vi "BS find all the buoys.vi"(0 "Image Src":T1, 1 "error in":errorcluster) -> (2 "Buoy Array":cluster{i16, i16}[](array[cluster]), 3 "Buoys found?":bool, 4 "error out":errorcluster)   [LabVIEW 2012]
doc: "This VI finds all the buoys and places there location into a 2D array. A valid flag is posted if completed."
uses:
  <vilib>/vision/Image Controls.llb/IMAQ Image.ctl
  <vilib>/vision/NI_Vision_Development_Module.lvlib
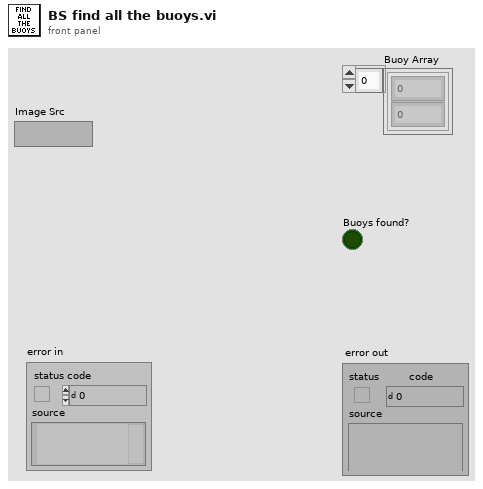
[diagram p1: front panel]
types:
  T1 = typedef "IMAQ Image.ctl" = refnum<image>
  T2 = enum32{"AutoM", "Close", "Dilate", "Erode", "Gradient", "Gradient in", "Gradient out", "HitMiss", "Open", "PClose", "POpen", "Thick", "Thin"}
  T3 = cluster{"Position":cluster{"x":sgl, "y":sgl}, "Angle":sgl, "Scale":sgl, "Score":sgl, "Bounding Box":cluster{"x":sgl, "y":sgl}[]}[]
  T4 = cluster{"Position":cluster{"x":sgl, "y":sgl}, "Angle":sgl, "Scale":sgl, "Score":sgl, "Bounding Box":cluster{"x":sgl, "y":sgl}[]}
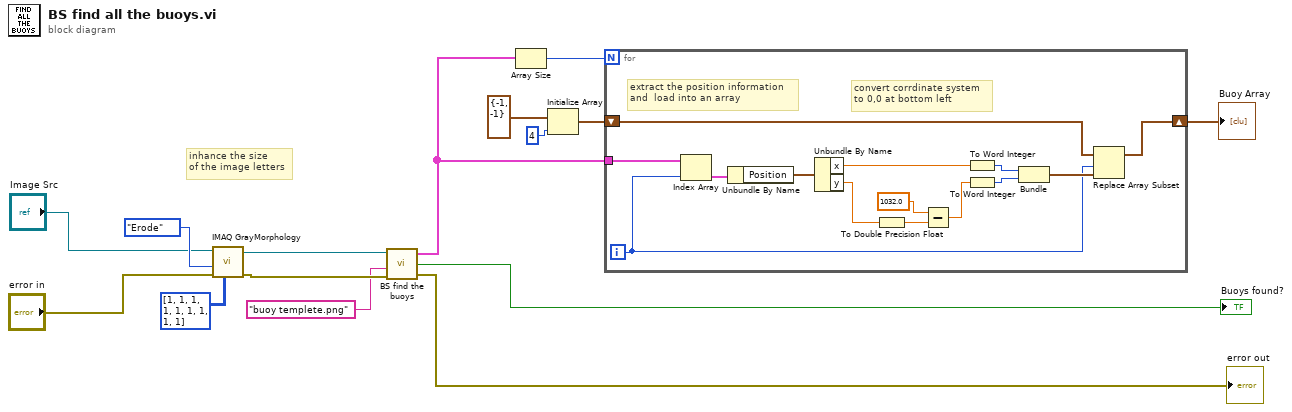
[diagram p0: block diagram]
diagram:
  # "inhance the size \nof the image letters"
  n1 = call "IMAQ GrayMorphology"("Structuring Element"=i32[][] [[1, 1, 1], [1, 1, 1], [1, 1, 1]] ("Structuring Element (Gray Morphology 1)"), "error in (no error)"="error in", "Operation"=T2."Erode" ("Operation (Gray Morphology 1)"), "Image Src"="Image Src") -> ("error out"=w10:errorcluster, "Image Dst Out"=w11:T1)  [unwired: 3 in, 3 out]
  n2 = call "BS find the buoys.vi"("Image Path"=w11, "templete path"="buoy templete.png", "error in"=w10) -> ("Matches"=w6:T3, "Valid?"=→"Buoys found?":bool, "error out"=→"error out":errorcluster)  [unwired: 2 in]
  n3 = Array Size(array=w6) -> (size(s)=w5:i32)
  n4 = Initialize Array(cluster{i16, i16} {-1, -1} ("buoy cluster"), 4 ("dimension size")) -> (w2:cluster{i16, i16}[])
  n5 = for {
    N: w5 -> [_]
    tunnel: w6 -> [w28]
    shift-right: [w20] -> w1
    shift-left: w2 -> [w23]
    i -> [w21]
    # "convert corrdinate system\nto 0,0 at bottom left"
    # "extract the position information\nand  load into an array"
    n6 = Index Array(array=w28, index=w21) -> (element=w29:T4)
    n7 = Unbundle By Name(w29) -> ("Position"=w26:cluster{"x":sgl, "y":sgl})
    n8 = Unbundle By Name(w26) -> ("x"=w27:sgl, "y"=w16:sgl)
    n9 = To Double Precision Float(number=w16) -> (double precision float=w17:dbl)
    n10 = Subtract(x=1032.0, y=w17) -> (x-y=w18:dbl)
    n11 = To Word Integer(number=w27) -> (16bit integer=w25:i16)
    n12 = To Word Integer(number=w18) -> (16bit integer=w24:i16)
    n13 = Bundle(w25, w24) -> (w22:cluster{i16, i16})  [unwired: 1 in]
    n14 = Replace Array Subset(array=w23, new element=w22, index=w21) -> (w20:cluster{i16, i16}[])
  }
  "Buoy Array" <- w1
